vi "_Remote Prepare Run 3 Data.vi"(6 "error in":errorcluster) -> (0 "error out":errorcluster, 1 "Steps":i32[][](array[numeric]), 2 "Scans":i32, 3 "Mass":dbl[][](array[numeric]), 4 "AcqMethod":T1[](array[typedef]) {"ScanType" format="%#.6g"; "Mass Range"."Res" items=["High/High", "Medium/Medium", "Low/Low", "High/Medium", "High/Low", "Medium/High", "Medium/Low", "Low/High", "Low/Medium"]}, 5 "Dwell":dbl[][](array[numeric]))   [LabVIEW 2015]
uses:
  Type/_XML Expt.ctl
  Type/_XML Lens.ctl
  Type/_Mass Range Property.ctl
  Type/_Mass Range Parameters.ctl
  Type/_RT Res Type.ctl
  Type/_RT Parameter.ctl
  Type/_RT Active Ch.ctl
  Type/_RT Expt.ctl
  Type/_Run Mode.ctl
  Type/_RT Mass Range.ctl
  Type/_File Type.ctl
  Type/_RT Command.ctl
  Configuration/_Global Configuration.vi
panel:
  # "(# of Expts) X (# of Masses)"
  # "(# of Expts) X (# of MassRanges)"
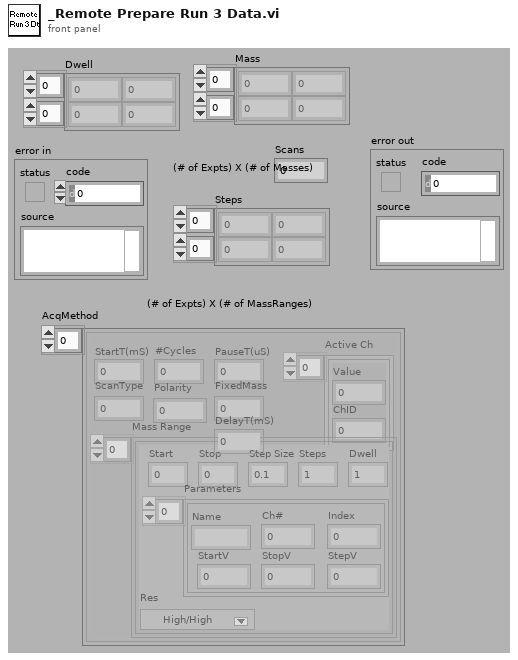
[diagram p1: front panel]
types:
  T1 = typedef "_XML Expt.ctl" = cluster{"StartT(mS)":i32, "#Cycles":i32, "PauseT(uS)":i32, "ScanType":i32, "Polarity":u8, "FixedMass":dbl, "DelayT(mS)":i32, "Active Ch":T2[], "Mass Range":T3[]}
  T2 = typedef "_XML Lens.ctl" = cluster{"Value":dbl, "ChID":u8}
  T3 = typedef "_Mass Range Property.ctl" = cluster{"Start":dbl, "Stop":dbl, "Step Size":dbl, "Steps":i32, "Dwell":dbl, "Parameters":T4[], "Res":T5}
  T4 = typedef "_Mass Range Parameters.ctl" = cluster{"Name":string, "Ch#":u8, "StartV":dbl, "StopV":dbl, "StepV":dbl, "Index":u8}
  T5 = typedef "_RT Res Type.ctl" = u16
  T6 = typedef "_RT Expt.ctl" = cluster{"StartT(mS)":i32, "#Cycles":i32, "Scan Type":T7, "PauseT(uS)":i32, "Polarity":u8, "DelayT(mS)":i32, "Active Ch":T8[], "Mass Range":T9[]}
  T7 = typedef "_Run Mode.ctl" = enum16{"MRM (Q1/Q2)", "Q1 Scan", "Q1 SRM", "Q2 Scan", "Q2 SRM", "Product Scan", "Precursor Scan", "Neutral Loss", "Neutral Gain"}
  T8 = typedef "_RT Active Ch.ctl" = cluster{"Start":i32, "Step":i32, "ChID":i32}
  T9 = typedef "_RT Mass Range.ctl" = cluster{"Steps":i32, "Dwell(uS)":i32, "Resolution Type":T5, "Ramping Ch":T8[]}
  T10 = typedef "_File Type.ctl" = enum16{"Configuration", "Old Configuration", "Calibration", "Resolution", "Diagnostic Method", "Old Method", "Acq Method", "Samp List"}
  T11 = typedef "_RT Parameter.ctl" = cluster{"RunMode":i32, "Initial Ch":T8[], "Sync":u8, "Expt":T6[], "EqTime(mS)":i32}
  T12 = typedef "_RT Command.ctl" = enum16{"Start", "StartActualRun", "Stop", "Runtime Update", "Get Data", "Get Info", "Get Status", "Get Param", "Get Config", "Get Table", "Read ADC", "Set Oscillator", "Update Config", "Update Table", "Set All Pol", "Set Pol and DC", "Set Max Mass", "Toggle RP", "Toggle EL", "Set PIC", "Initialize Turbo", "Send Turbo Comm", "Close Turbo", "P1", "P2", "P3", "Send Serial", "Set LC Out", "Get LC In", "Read VAC", "Test Table", "Toggle Power", "Get Startup", "Set Startup", "Get ADC Table", "Set ADC Table", "Get Brief Status", "Get Detail Status", "Auxiliary Update", "Set CC Logics", "Set CC Input Logics", "Ignore Error"}
  T13 = typedef "_RT Configuration 2.ctl" = cluster{"Name":string, "Ch#":u8, "Min":dbl, "Max":dbl, "Def+":dbl, "Def-":dbl, "Offset":dbl, "Slope":dbl, "Type":u8, "Description":string, "SettleT":dbl}
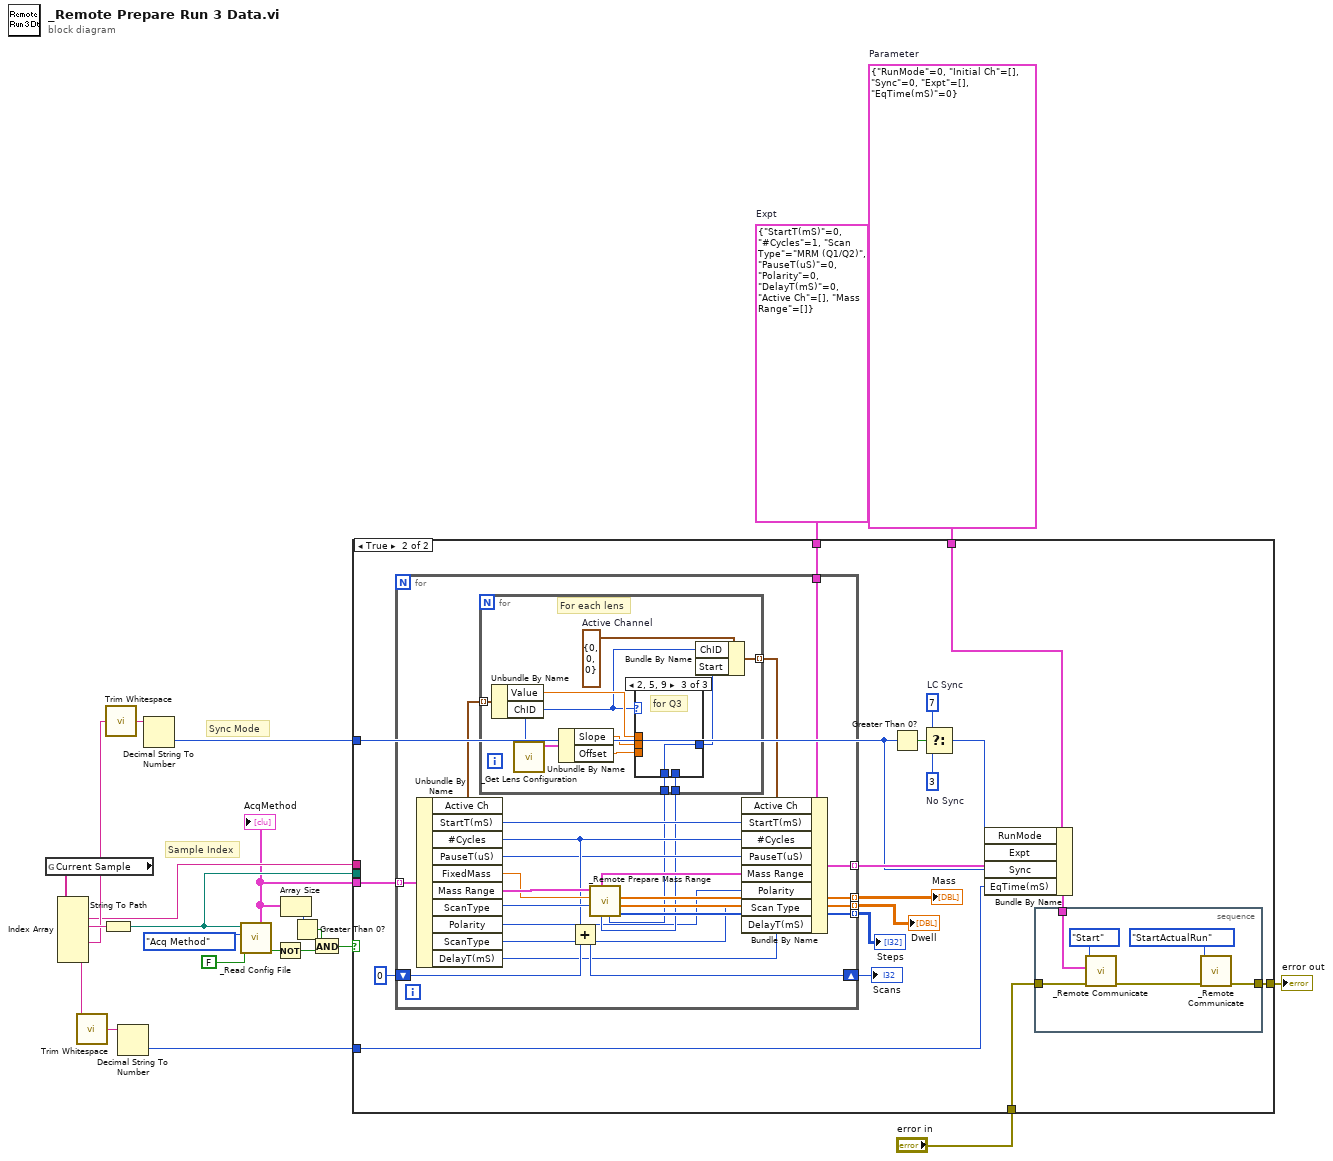
[diagram p0: block diagram]
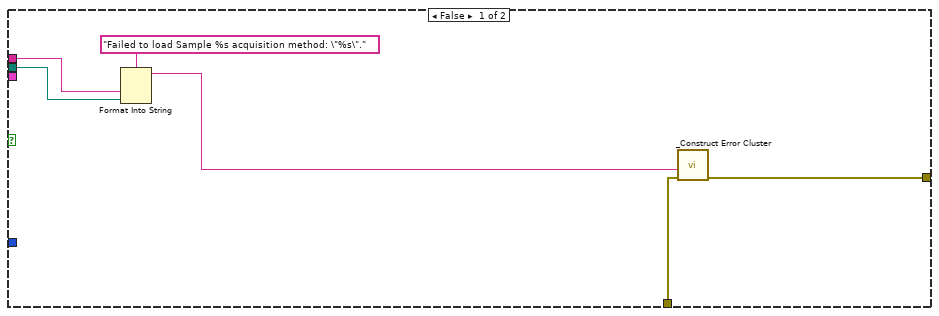
[diagram p2: hidden frame]
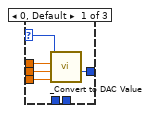
[diagram p3: hidden frame]
diagram:
  w11 = T6 {"StartT(mS)"=0, "#Cycles"=1, "Scan Type"=enum."MRM (Q1/Q2)", "PauseT(uS)"=0, "Polarity"=0, "DelayT(mS)"=0, "Active Ch"=[], "Mass Range"=[]}  # Expt
  w10 = T11 {"RunMode"=0, "Initial Ch"=[], "Sync"=0, "Expt"=[], "EqTime(mS)"=0}  # Parameter
  # "Sample Index"
  # "Sync Mode"
  n1 = global read "_Global Configuration.vi" "Current Sample"() -> (w21:string[])
  n2 = Index Array(array=w21) -> (element #1=w7:string, element #2=w20:string, element #4=w19:string, element #6=w2:string)  [unwired: 6 in, 2 out]
  n3 = call <vilib>:"Trim Whitespace.vi"("string"=w2) -> ("trimmed string"=w3:string)  [unwired: 1 in]
  n4 = String To Path(string=w20) -> (path=w6:path)
  n5 = call <vilib>:"Trim Whitespace.vi"("string"=w19) -> ("trimmed string"=w22:string)  [unwired: 1 in]
  n6 = Decimal String To Number(string=w3) -> (number=w1:i32)  [unwired: 3 out]
  n7 = Decimal String To Number(string=w22) -> (number=w4:i32)  [unwired: 3 out]
  n8 = call "_Read Config File.vi"("advisory dialog? (display:T)"=FALSE, "File Type (config)"=_File_Type."Acq Method", "start path  (Not A Path)"=w6) -> ("error"=w14:bool, "AcqMethod"=w5:T1[])  [unwired: 7 out]
  "AcqMethod" <- w5
  n9 = Not(x=w14) -> (.not. x?=w13:bool)
  n10 = Array Size(array=w5) -> (size(s)=w16:i32)
  n11 = Greater Than 0?(x=w16) -> (x > 0?=w15:bool)
  n12 = And(x=w15, y=w13) -> (x .and. y?=w12:bool)
  n13 = case shown="True" w12 {
    tunnel: w5 -> [_ w38]
    tunnel: w11 -> [_ w46]
    tunnel: w10 -> [_ w44]
    tunnel: [w27 w36] -> w8
    tunnel: "error in" -> [w28 w30]
    tunnel: w7 -> [w26 _]
    tunnel: w6 -> [w25 _]
    tunnel: w4 -> [_ w31]
    tunnel: w1 -> [_ w29]
    frame False {
      n14 = Format Into String(format string="Failed to load Sample %s acquisition method: \"%s\".", w26, w25) -> (resulting string=w23:string)  [unwired: 2 in, 1 out]
      n15 = call "_Construct Error Cluster.vi"("error in"=w28, "reason"=w23) -> ("error out"=w27:errorcluster)  [unwired: 2 in, 3 out]
    }
    frame True {
      w34 = 3  # No Sync
      w35 = 7  # LC Sync
      n16 = for {
        tunnel: w38 -> [w74] mode=indexing
        tunnel: [w70] -> w40 mode=indexing
        tunnel: [w69] -> w41 mode=indexing
        tunnel: [w68] -> w42 mode=indexing
        shift-right: [w66] -> w43
        shift-left: 0 -> [w67]
        tunnel: w46 -> [w65]
        tunnel: [w56] -> w45 mode=indexing
        n17 = Unbundle By Name(w74) -> ("Active Ch"=w60:T2[], "StartT(mS)"=w62:i32, "#Cycles"=w63:i32, "PauseT(uS)"=w61:i32, "FixedMass"=w72:dbl, "Mass Range"=w73:T3[], "ScanType"=w71:i32, "Polarity"=w55:u8, "ScanType"=w54:i32, "DelayT(mS)"=w53:i32)
        n18 = Add(x=w63, y=w67) -> (x+y=w66:i32)
        n19 = call "_Remote Prepare Mass Range.vi"("Run Mode"=w71, "Fixed Mass (amu)"=w72, "GUI Mass Ranges"=w73) -> ("Steps"=w68:i32[], "Dwell (ms)"=w69:dbl[], "Mass"=w70:dbl[], "Init Q2 Mass"=w57:i32, "Init Q1 Mass"=w58:i32, "RT Mass Ranges"=w64:T9[])  [unwired: 3 out]
        n20 = for {
          tunnel: [w81] -> w59 mode=indexing
          tunnel: w60 -> [w80] mode=indexing
          tunnel: w58 -> [w76]
          tunnel: w57 -> [w75]
          w83 = T8 {"Start"=0, "Step"=0, "ChID"=0}  # Active Channel
          # "For each lens"
          n21 = Unbundle By Name(w80) -> ("Value"=w79:dbl, "ChID"=w78:u8)
          n22 = call "_Get Lens Configuration.vi"("Channel #"=w78) -> ("Lens Configuration"=w77:T13)  [unwired: 1 in, 5 out]
          n23 = Unbundle By Name(w77) -> ("Slope"=w85:dbl, "Offset"=w84:dbl)
          n24 = case shown="2, 5, 9" w78 {
            selector: w78 -> [w86 _ _]
            tunnel: w79 -> [w90 _ _]
            tunnel: w85 -> [w89 _ _]
            tunnel: w84 -> [w88 _ _]
            tunnel: [w87 w91 w92] -> w82
            tunnel: w76 -> [_ w91 _]
            tunnel: w75 -> [_ _ w92]
            frame 0, Default {
              n25 = call "_Convert to DAC Value.vi"("Offset"=w88, "Slop"=w89, "Number"=w90, "Channel"=w86) -> ("DAC Value"=w87:i32)  [unwired: 2 in, 5 out]
            }
            frame 1, 4, 7 {
              # "for Q1"
            }
            frame 2, 5, 9 {
              # "for Q3"
            }
          }
          n26 = Bundle By Name(cluster=w83, "ChID"=w78, "Start"=w82) -> (w81:T8)
        }
        n27 = Bundle By Name(cluster=w65, "Active Ch"=w59, "StartT(mS)"=w62, "#Cycles"=w63, "PauseT(uS)"=w61, "Mass Range"=w64, "Polarity"=w55, "Scan Type"=w54, "DelayT(mS)"=w53) -> (w56:T6)
      }
      "Scans" <- w43
      "Steps" <- w42
      "Dwell" <- w41
      "Mass" <- w40
      n28 = Greater Than 0?(x=w31) -> (x > 0?=w33:bool)
      n29 = Select(t=w35, s=w33, f=w34) -> (s? t:f=w32:i32)
      n30 = Bundle By Name(cluster=w44, "RunMode"=w32, "Expt"=w45, "Sync"=w31, "EqTime(mS)"=w29) -> (w37:T11)
      n31 = stacked-sequence {
        tunnel: w37 -> [w51]
        tunnel: [w47] -> w36
        tunnel: w30 -> [w50]
        frame #0 {
          n32 = call "_Remote Communicate.vi"("error in (no error)"=w50, "Parameter"=w51, "Command"=_RT_Command."Start") -> ("error out"=w48:errorcluster)  [unwired: 3 in, 3 out]
          n33 = call "_Remote Communicate.vi"("error in (no error)"=w48, "Command"=_RT_Command."StartActualRun") -> ("error out"=w47:errorcluster)  [unwired: 4 in, 3 out]
        }
      }
    }
  }
  "error out" <- w8
